vi "Write Raw Data Queue.vi"(8 "error in (no error)":errorcluster, 11 "output waveform":waveform(cdb)) -> (0 "error out":errorcluster)   [LabVIEW 2016]
uses:
  Application Control/Application Globals.vi
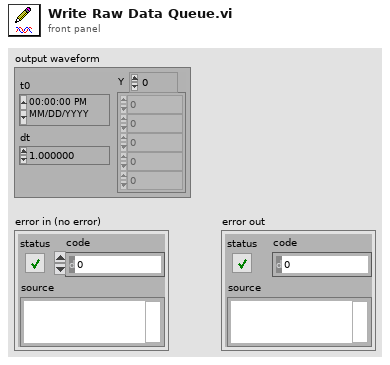
[diagram p1: front panel]
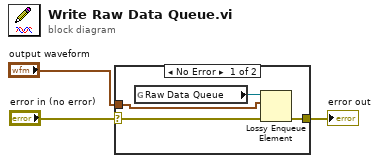
[diagram p0: block diagram]
diagram:
  n1 = case shown="No Error" "error in (no error)" {
    selector: "error in (no error)" -> [w7 w8]
    tunnel: "output waveform" -> [w5 _]
    tunnel: [w4 w8] -> w3
    frame No Error {
      n2 = global read "Application Globals.vi" "Raw Data Queue"() -> (w6:refnum<queue>)
      n3 = Lossy Enqueue Element(queue=w6, element=w5, error in (no error)=w7) -> (error out=w4:errorcluster)  [unwired: 3 out]
    }
    frame Error {
    }
  }
  "error out" <- w3
